vi "Test high resolution sleep.vi"() -> ()   [LabVIEW 2021]
uses:
  Time Conversion/LabVIEW Time to UTC Time.vi
  CIFCore/Common/Utilities/Add Error.vi
  CIFCore/Common/Utilities/Append Error Location.vi
  CIFClocks.lvlib
  <vilib>/NI_Real-Time Target Support.lvlib
panel:
  out "Array":cluster{dbl, dbl, dbl, dbl}[](array[cluster])
  in  "stop":bool
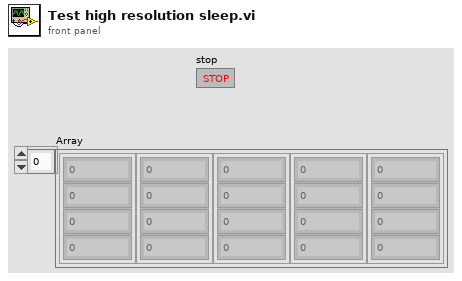
[diagram p1: front panel]
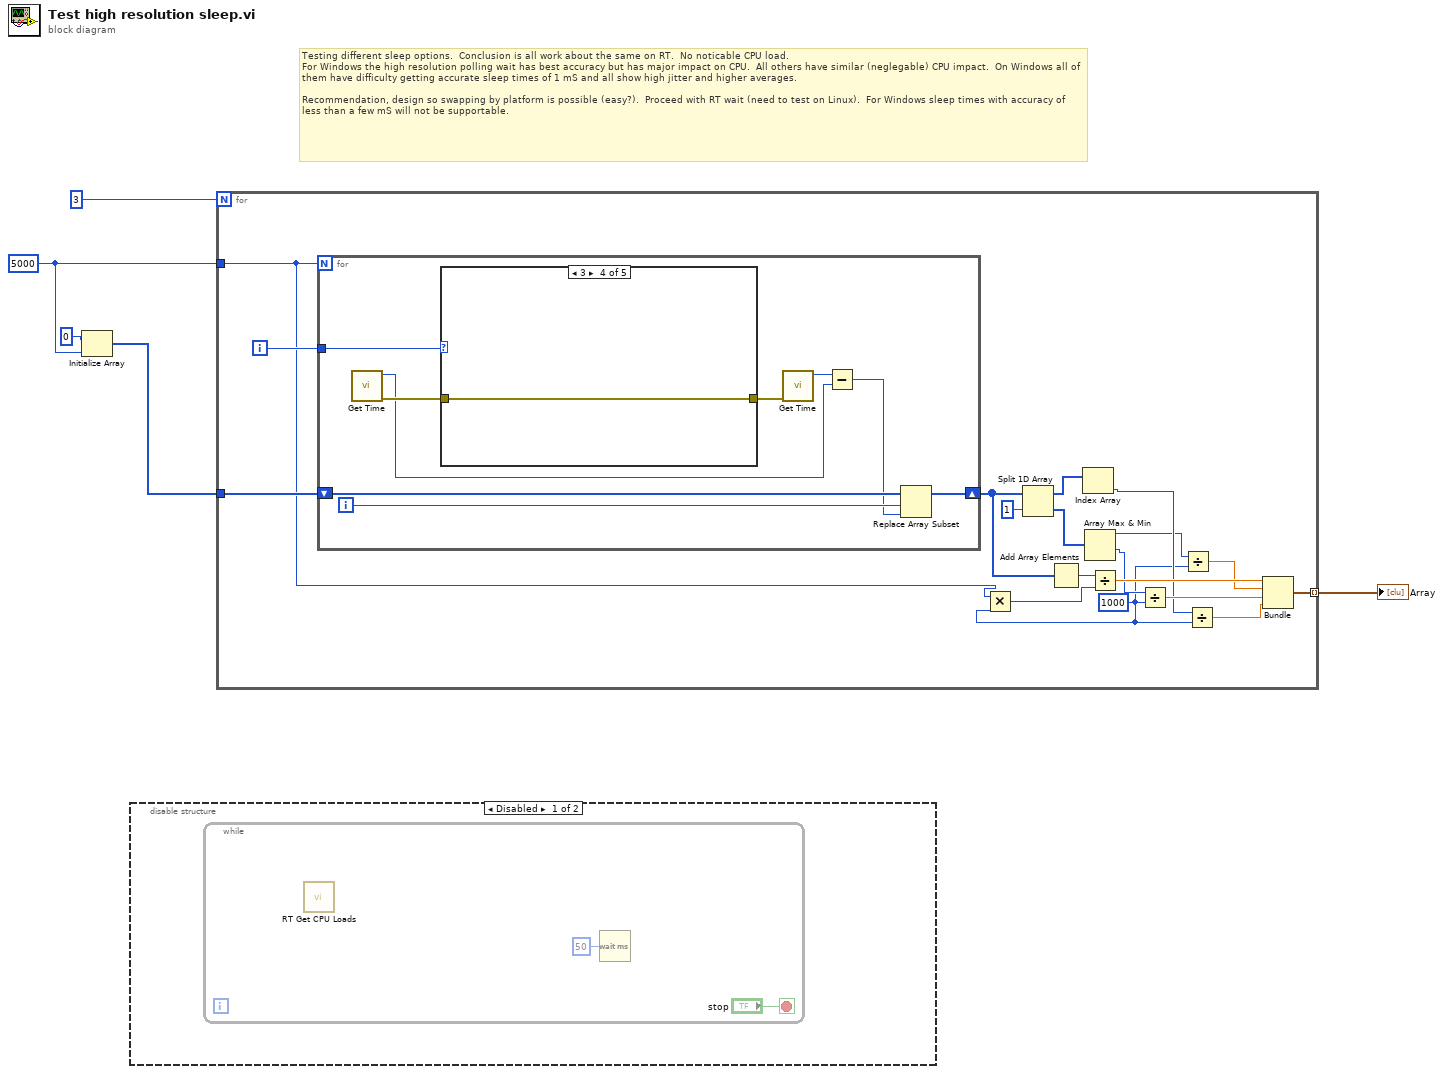
[diagram p0: block diagram]
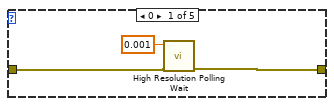
[diagram p2: hidden frame]
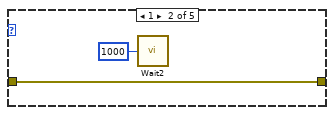
[diagram p3: hidden frame]
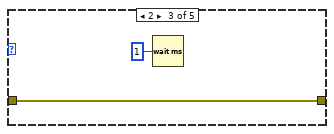
[diagram p4: hidden frame]
diagram:
  w4 = 5000
  # "Testing different sleep options.  Conclusion is all work about the same on RT.  No noticable CPU load.\nFor Windows the high resolution polling wait has best accuracy but has major impact on CPU.  All others have similar (neglegable) CPU impact.  On Windows all of them have difficulty getting accurate sleep times of 1 mS and all show high jitter and higher averages.  \n\nRecommendation, design so swapping by platform is possible (easy?).  Proceed with RT wait (need to test on Linux).  For Windows sleep times with accuracy of less than a few mS will not be supportable."
  n1 = Initialize Array(u64 0, w4) -> (w2:u64[])
  n2 = disable-structure shown="Disabled" {
    frame Disabled {
      n3 = while {
        stop <- "stop" stop-if-true
        n4 = call <vilib>:"RT Get CPU Loads.vi"() -> ()  [unwired: 10 in, 2 out]
        n5 = Wait (ms)(milliseconds to wait=u32 50) -> ()  [unwired: 1 out]
      }
    }
    frame Enabled {
    }
  }
  n6 = for {
    N: 3 -> [_]
    tunnel: w4 -> [w10]
    tunnel: w2 -> [w24]
    tunnel: [w23] -> w1 mode=indexing
    i -> [w25]
    w8 = u64 1000 ("y")
    n7 = for {
      N: w10 -> [_]
      tunnel: w25 -> [w30]
      shift-right: [w28] -> w19
      shift-left: w24 -> [w29]
      i -> [w27]
      n8 = call "Get Time.vi"() -> ("error out"=w34:errorcluster, "Time (ns)"=w31:u64)  [unwired: 9 in, 1 out]
      n9 = case shown="3" w30 {
        tunnel: w34 -> [w36 w39 w40 w42 w43]
        tunnel: [w35 w39 w40 w42 w43] -> w33
        frame 0 {
          n10 = call <vilib>:"High Resolution Polling Wait.vi"("error in (no error)"=w36, "seconds to wait"=0.001) -> ("error out"=w35:errorcluster)  [unwired: 9 in]
        }
        frame 1 {
          n11 = call "Wait2"("Count(uSec)"=u32 1000) -> ()  [unwired: 1 out]
        }
        frame 2 {
          n12 = Wait (ms)(milliseconds to wait=u32 1) -> ()  [unwired: 1 out]
        }
        frame 3 {
        }
        frame 100, Default {
        }
      }
      n13 = call "Get Time.vi"("error in (no error)"=w33) -> ("Time (ns)"=w32:u64)  [unwired: 8 in, 2 out]
      n14 = Subtract(x=w32, y=w31) -> (x-y=w26:u64)
      n15 = Replace Array Subset(array=w29, new element=w26, index=w27) -> (w28:u64[])
    }
    n16 = Multiply(x=w10, y=w8) -> (x*y=w9:u64)
    n17 = Split 1D Array(array=w19, index=1) -> (first subarray=w21:u64[], second subarray=w20:u64[])
    n18 = Add Array Elements(numeric array=w19) -> (sum=w18:u64)
    n19 = Index Array(array=w21) -> (element=w14:u64)  [unwired: 1 in]
    n20 = Array Max & Min(array=w20) -> (max value=w12:u64, min value=w16:u64)  [unwired: 2 out]
    n21 = Divide(x=w18, y=w9) -> (x/y=w17:dbl)
    n22 = Divide(x=w16, y=w8) -> (x/y=w15:dbl)
    n23 = Divide(x=w12, y=w8) -> (x/y=w11:dbl)
    n24 = Divide(x=w14, y=w8) -> (x/y=w13:dbl)
    n25 = Bundle(w17, w11, w15, w13) -> (w23:cluster{dbl, dbl, dbl, dbl})  [unwired: 1 in]
  }
  "Array" <- w1
